vi "Try Beta Version of CSMF.vi"() -> ()   [LabVIEW 2017]
uses:
  <vilib>/JKI/VIPM API/command-line/support/Library Contents Cluster_vipm_api.ctl
  _Try Beta Version of CSMF/_Try Beta Version of CSMF.lvlib
  <vilib>/JKI/VIPM API/VIPM API_vipm_api.lvlib
panel:
  out "Next Actions":string
  out "Information":string
  # "Warning: You should login VIPM and change it to community/Pro edtion firstly."
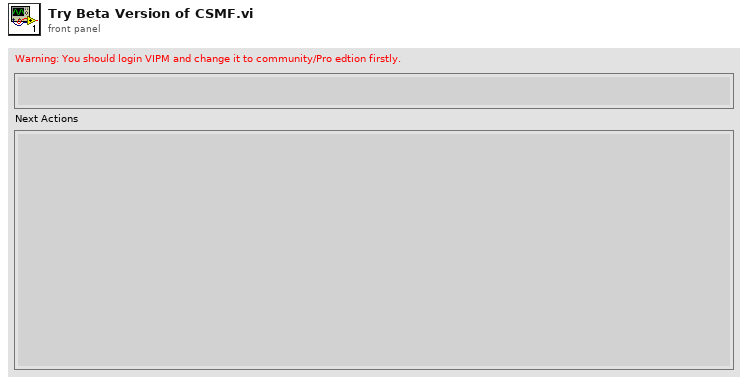
[diagram p1: front panel]
types:
  T1 = enum32{"Invalid", "Standard", "Closed", "Hidden", "Minimized", "Maximized"}
  T2 = enum32{"invalid app kind", "Development System", "Run Time System", "Student Edition", "Embedded LabVIEW", "Evaluation", "Custom"}
  T3 = enum16{"open", "replace", "create", "open or create", "replace or create", "replace or create with confirmation"}
  T4 = typedef "VIPM API_vipm_api.lvlib/Library Contents Cluster_vipm_api.ctl" = cluster{"Package Name":string, "Version":string, "Display Name":string, "Repository Name":string, "Company Name":string, "License Type":string, "Installed":bool, "Deprecated":bool, "Dependency or Conflict Problem":bool, "Downloaded":bool}
  T5 = cluster{"Core":cluster{"Current VI Reference":refnum<vi>, "Close Panel on Exit?":bool}, "ftpInfo":cluster{"address":string, "remote port (21)":u16, "userName":string, "passWord":string}, "CSMF":string[], "Library[]":T4[], "CSMFTempPath":path[]}
  T6 = cluster{"address":string, "remote port (21)":u16, "userName":string, "passWord":string}
  T7 = cluster{"Current VI Reference":refnum<vi>, "Close Panel on Exit?":bool}
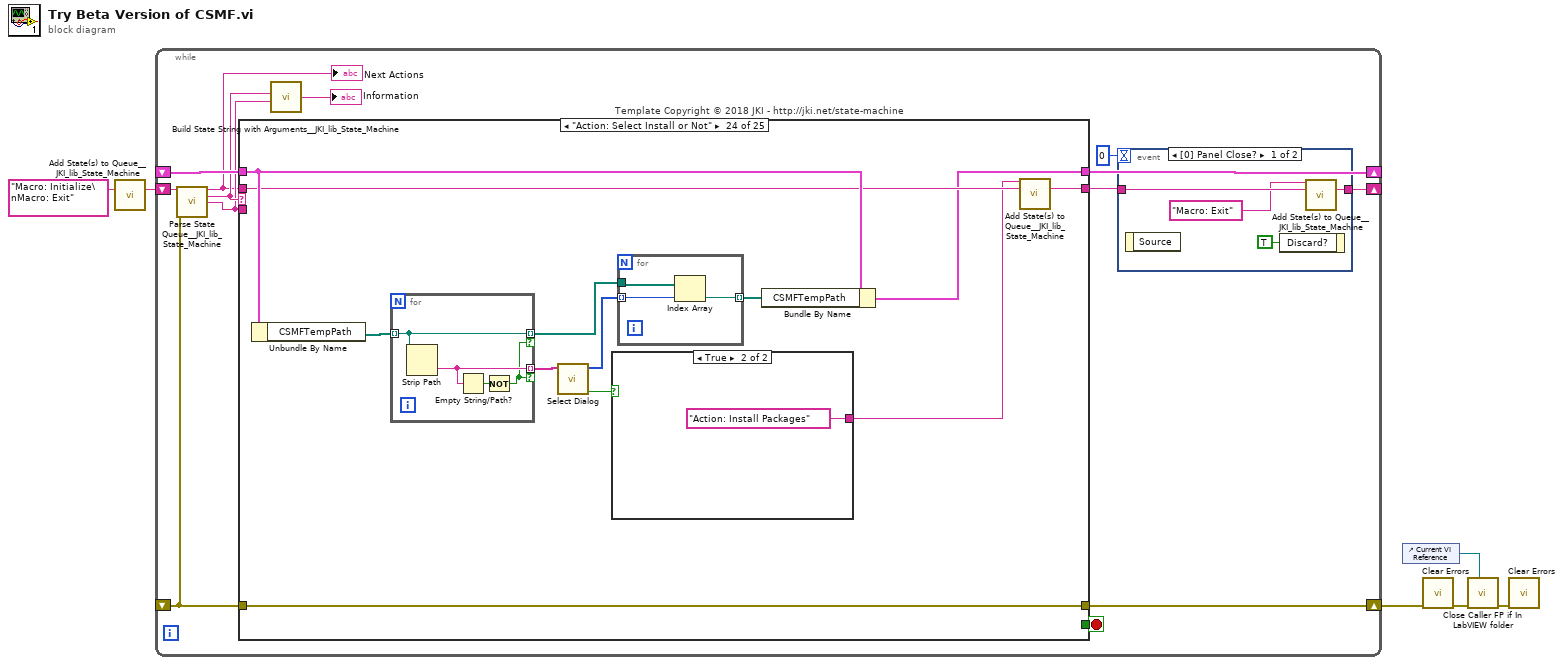
[diagram p0: block diagram]
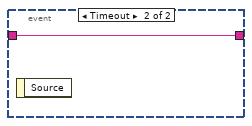
[diagram p2: hidden frame]
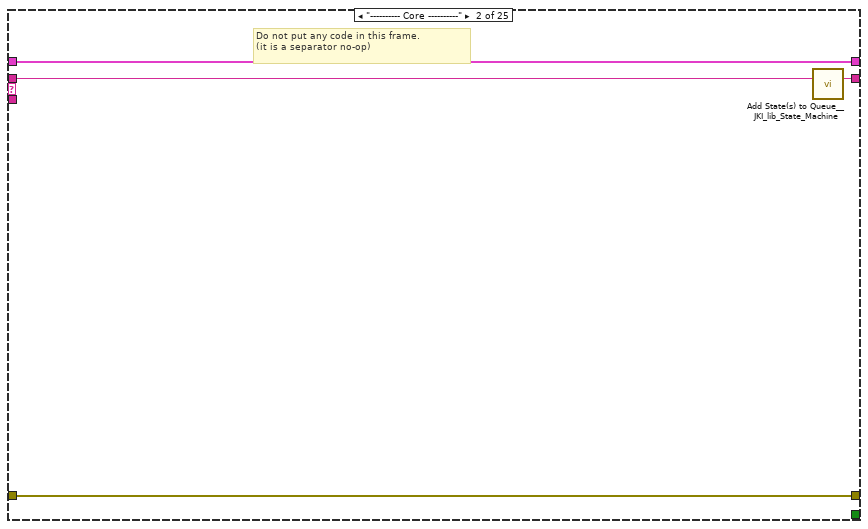
[diagram p4: hidden frame]
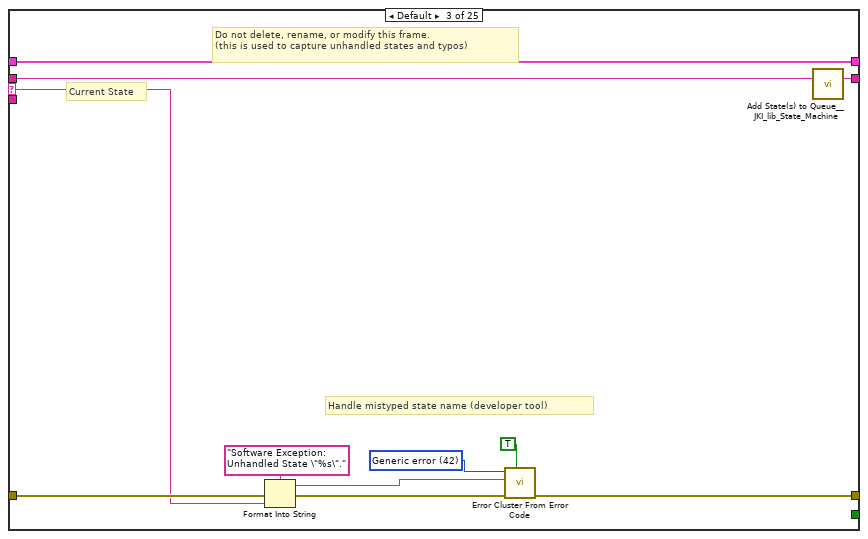
[diagram p5: hidden frame]
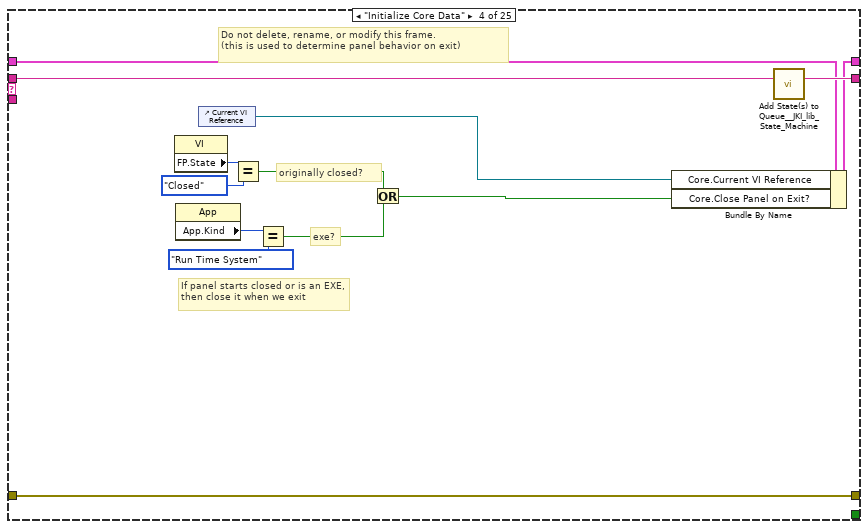
[diagram p6: hidden frame]
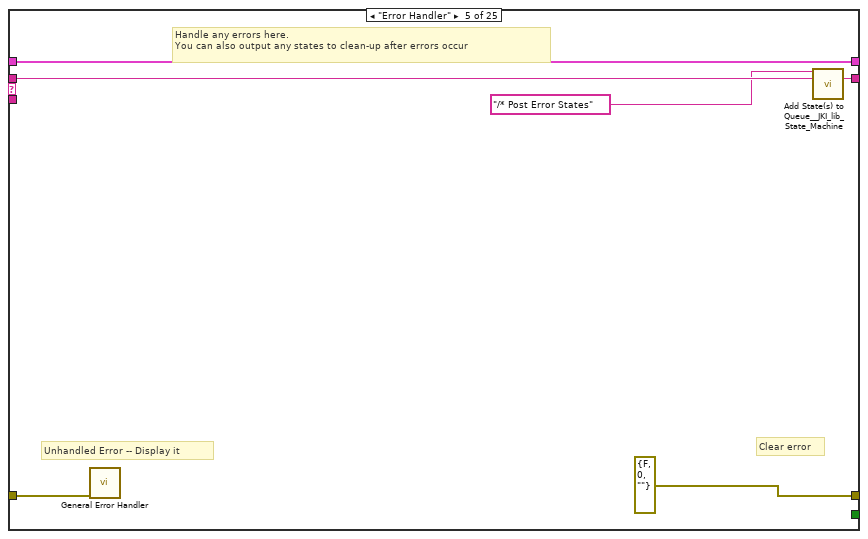
[diagram p7: hidden frame]
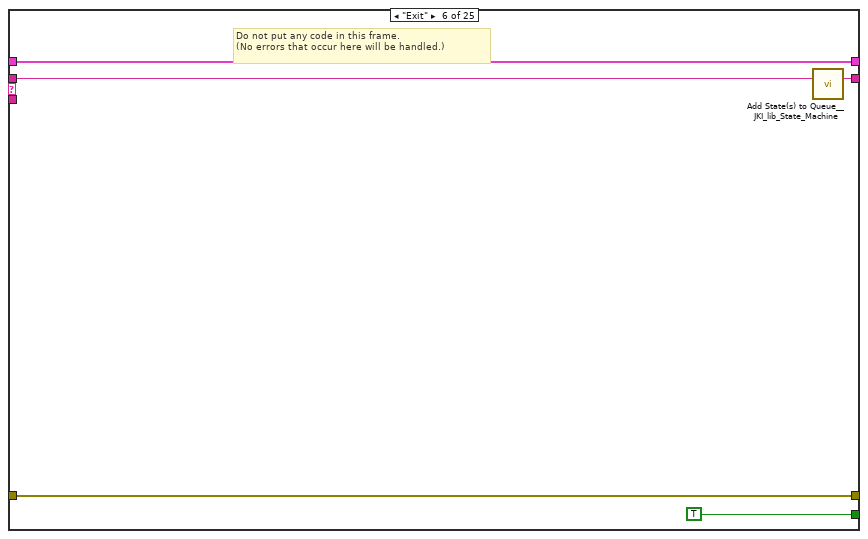
[diagram p8: hidden frame]
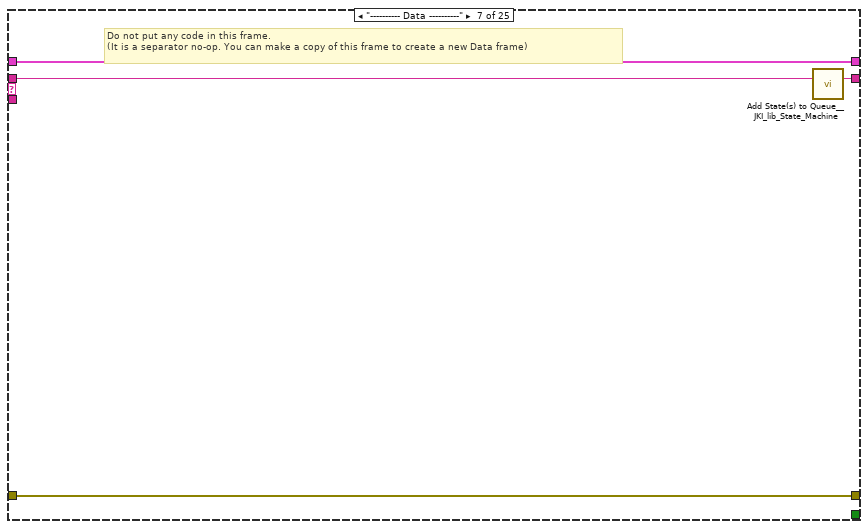
[diagram p9: hidden frame]
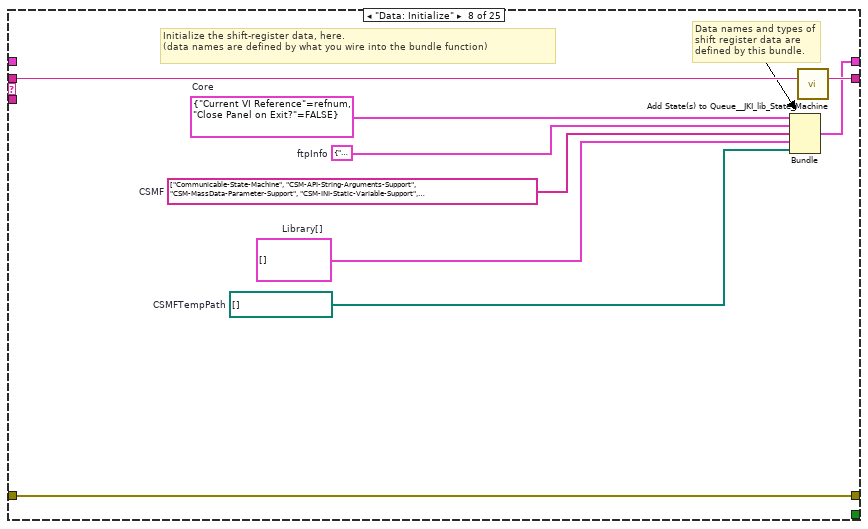
[diagram p10: hidden frame]
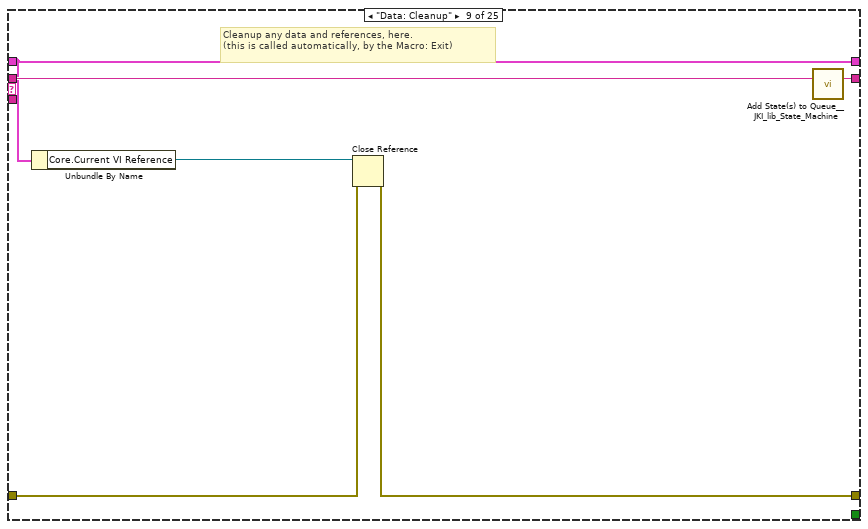
[diagram p11: hidden frame]
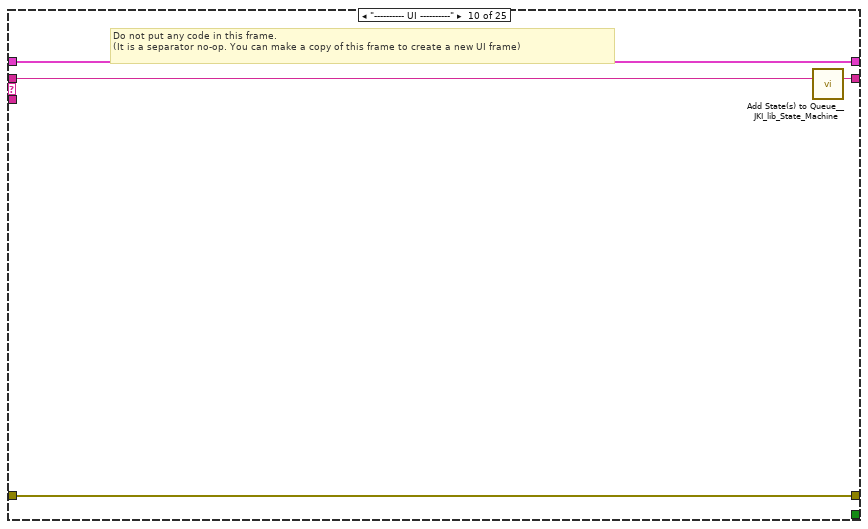
[diagram p12: hidden frame]
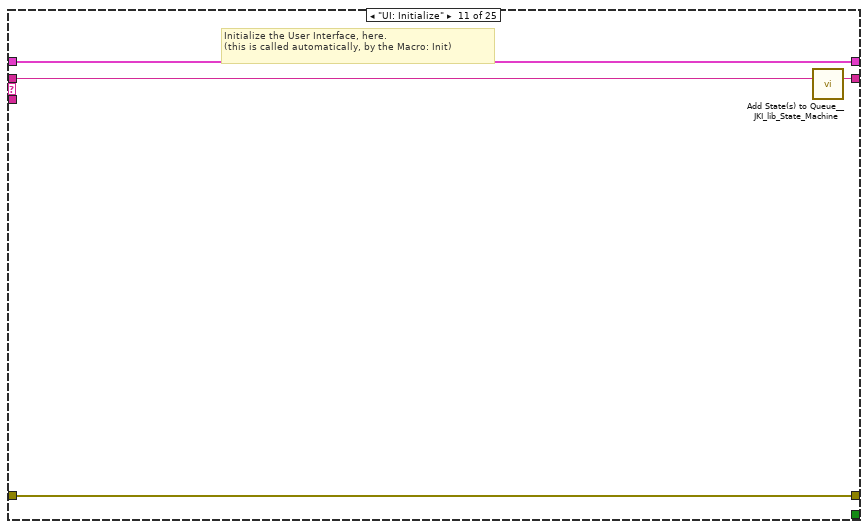
[diagram p13: hidden frame]
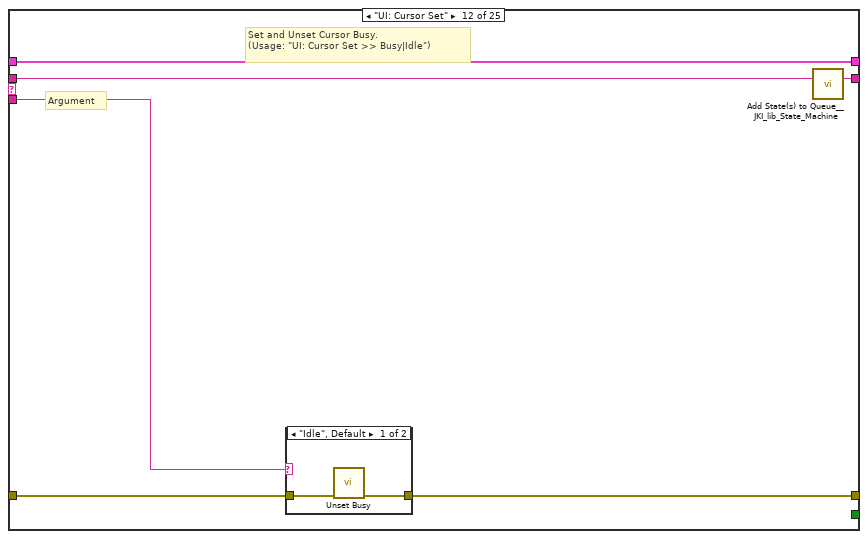
[diagram p14: hidden frame]
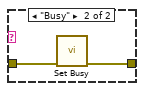
[diagram p15: hidden frame]
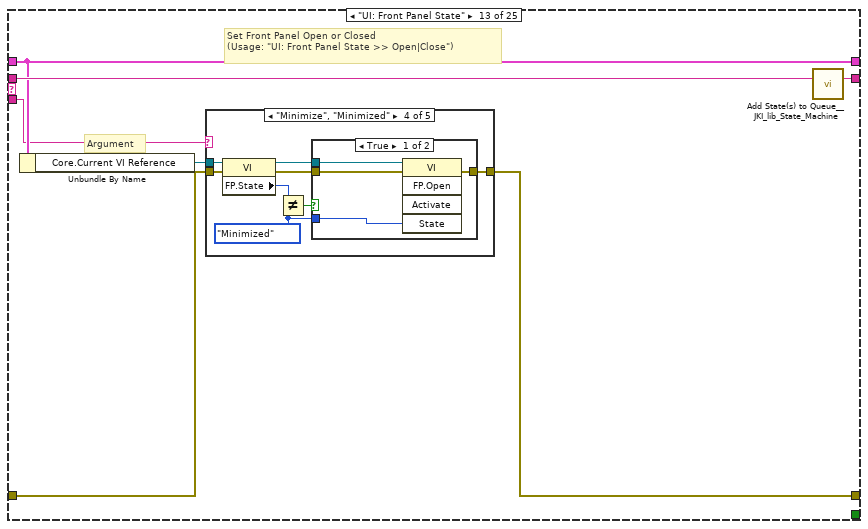
[diagram p16: hidden frame]
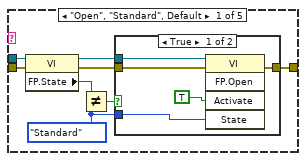
[diagram p17: hidden frame]
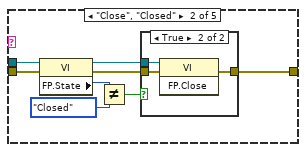
[diagram p19: hidden frame]
diagram:
  n1 = call <vilib>:"Add State(s) to Queue__JKI_lib_State_Machine.vi"("State(s) in (\"\")"="Macro: Initialize\nMacro: Exit") -> ("States Out"=w3:string)  [unwired: 14 in]
  n2 = while {
    shift-right: [w16] -> _
    shift-left: _ -> [w15]
    shift-right: [w18] -> w2
    shift-left: _ -> [w14]
    shift-right: [w8] -> _
    shift-left: w3 -> [w19]
    stop <- w17 stop-if-true
    # "Template Copyright © 2018 JKI - http://jki.net/state-machine"
    n3 = call <vilib>:"Parse State Queue__JKI_lib_State_Machine.vi"("State Queue"=w19, "Error In (no error)"=w14) -> ("Remaining States"=w10:string, "Current State"=w13:string, "Arguments"=w11:string)  [unwired: 11 in]
    "Next Actions" <- w10
    n4 = case shown="\"Action: Select Install or Not\"" w13 {
      selector: w13 -> [_ _ w32 _ _ _ _ _ _ _ _ _ _ _ _ _ _ _ _ _ _ _ _ _ _]
      tunnel: w10 -> [w27 w31 w36 w55 w61 w66 w70 w79 w85 w89 w93 w99 w110 w179 w184 w189 w207 w211 w225 w231 w241 w247 w254 w263 w287]
      tunnel: w11 -> [_ _ _ _ _ _ _ _ _ _ _ w94 w104 _ _ _ _ _ _ _ w238 _ _ _ _]
      tunnel: w15 -> [w25 w28 w34 w48 w58 w64 w67 _ w80 w86 w91 w97 w106 w176 w181 w186 w204 w208 w216 w228 w240 w250 w253 w265 w286]
      tunnel: [w26 w29 w38 w52 errorcluster {"status"=FALSE, "code"=0, "source"=""} ("error out") w63 w68 w76 w81 w87 w90 w95 w107 w177 w182 w192 w205 w209 w223 w229 w234 w249 w251 w266 w275] -> w18
      tunnel: w14 -> [w26 w29 w37 w52 w57 w63 w68 w76 w82 w87 w90 w96 w108 w177 w182 w192 w205 w209 w223 w229 _ _ _ w266 _]
      tunnel: [w27 w30 w35 w54 w60 w65 w69 w78 w84 w88 w92 w98 w109 w178 w183 w190 w206 w210 w224 w230 w241 w248 w254 w264 w287] -> w9
      tunnel: [_ _ _ _ _ TRUE _ _ _ _ _ _ _ _ _ _ _ _ _ _ _ _ _ _ _] -> w17
      tunnel: [w25 w28 w34 w53 w58 w64 w67 w77 w80 w86 w91 w97 w106 w176 w181 w186 w204 w208 w214 w227 w236 w250 w253 w259 w278] -> w16
      frame "", "Event Structure", "Idle" {
        # "executes when the state queue is empty"
      }
      frame "---------- Core ----------" {
        # "Do not put any code in this frame.\n(it is a separator no-op)"
        n5 = call <vilib>:"Add State(s) to Queue__JKI_lib_State_Machine.vi"("State(s) in (\"\")"=w31) -> ("States Out"=w30:string)  [unwired: 14 in]
      }
      frame Default {
        w41 = 42 items=["No error", "Argument error", "Memory is full", "Out of zone", "End of file", "File already open", "Generic file I/O error", "File not found", "File permission error", "Disk is full", "Duplicate path", "Too many files open", "System feature not enabled", "Resource file not found", "Cannot add resource", "Resource not found", "Image not found", "Image memory error", "Pen does not exist", "Config type invalid", "Config token not found", "Config parse error", "Config memory error", "Bad external code format", "Bad external code offset", "External code not present", "Null window", "Destroy window error", "Null menu", "Print aborted", "Bad print record", "Print driver error", "Windows error during printing", "Memory error during printing", "Print dialog error", "Generic print error", "Invalid device refnum", "Device not found", "Device parameter error", "Device unit error", "Cannot open device", "Device call aborted", "Generic error", "Cancelled by user", "Object ID too low", "Object ID too high", "Object not in heap", "Unknown heap", "Unknown object (invalid DefProc)", "Unknown object (DefProc not in table)", "Message out of range", "Invalid (null) method", "Unknown message", "Manager call not supported", "Bad address", "Network operation in progress", "Network operation timed out", "Connection is busy", "Network attribute not supported", "Network error", "Address in use", "System out of memory", "Connection aborted", "Connection refused", "Not connected", "Already connected", "Connection closed", "Initialization error (interapplication manager)", "Bad occurrence", "Wait on unbound occurrence handler", "Occurrence queue overflow", "Datalog type conflict", "Unused", "Unrecognized type (interapplication manager)", "Memory corrupt", "Failed to make temporary DLL", "Old CIN version", "Drag socket not found", "Failed to load drop-object", "Failed to register OLE object", "Failed to release OLE object", "Format specifier type mismatch", "Unknown format specifier", "Too few format specifiers", "Too many format specifiers", "Scan failed", "Newer CIN version", "Error converting to variant", "Runtime menu error", "Password tampered", "Variant attribute not found", "Incompatible variant data type", "Event data is not available", "Event Store is not present", "Occurrence is not found", "Event Queue is not created", "Event info is not available", "Refnum passed is NULL", "Error retrieving Class GUID", "Error retrieving CoClass GUID", "Error retrieving TypeLib GUID.", "Bad built application magic bytes.", "Specific driver is different from the specific driver associated with the Logical Name.", "There is no session opened to the class driver.", "Max Error", "MAX - Error with config objects", "MAX - Error loading configuration", "MAX - Group not supported"]
        # "Current State"
        # "Do not delete, rename, or modify this frame.\n(this is used to capture unhandled states and typos)"
        # "Handle mistyped state name (developer tool)"
        n6 = Format Into String(format string="Software Exception: Unhandled State \"%s\"." ("message"), error in=w37, w32) -> (resulting string=w40:string, error out=w39:errorcluster)  [unwired: 1 in]
        n7 = call <vilib>:"Error Cluster From Error Code.vi"("show call chain? (False)"=TRUE, "error in (no error)"=w39, "error message (\"\")"=w40, "error code (0)"=w41) -> ("error out"=w38:errorcluster)  [unwired: 5 in]
        n8 = call <vilib>:"Add State(s) to Queue__JKI_lib_State_Machine.vi"("State(s) in (\"\")"=w36) -> ("States Out"=w35:string)  [unwired: 14 in]
      }
      frame "Initialize Core Data" {
        # "Do not delete, rename, or modify this frame.\n(this is used to determine panel behavior on exit)"
        # "originally closed?"
        # "exe?"
        # "If panel starts closed or is an EXE, then close it when we exit"
        n9 = property class="VI"() -> ("FP.State"=w45:T1)  [unwired: 2 in, 2 out]
        n10 = property class="App"() -> ("App.Kind"=w51:T2)  [unwired: 2 in, 2 out]
        n11 = control-ref of="Current VI Reference"() -> (w46:refnum<vi>)
        n12 = Equal?(x=w45, y=T1."Closed" ("Front Panel Window:State")) -> (x = y?=w43:bool)
        n13 = Equal?(x=w51, y=T2."Run Time System" ("Application:Kind")) -> (x = y?=w49:bool)
        n14 = Or(x=w43, y=w49) -> (x .or. y?=w47:bool)
        n15 = Bundle By Name(cluster=w48, "Core.Current VI Reference"=w46, "Core.Close Panel on Exit?"=w47) -> (w53:T5)
        n16 = call <vilib>:"Add State(s) to Queue__JKI_lib_State_Machine.vi"("State(s) in (\"\")"=w55) -> ("States Out"=w54:string)  [unwired: 14 in]
      }
      frame "Error Handler" {
        # "Unhandled Error -- Display it"
        # "Handle any errors here.\nYou can also output any states to clean-up after errors occur"
        # "Clear error"
        n17 = call <vilib>:"General Error Handler.vi"("error in (no error)"=w57) -> ()  [unwired: 10 in, 5 out]
        n18 = call <vilib>:"Add State(s) to Queue__JKI_lib_State_Machine.vi"("State(s) in Front (\"\")"="/* Post Error States", "State(s) in (\"\")"=w61) -> ("States Out"=w60:string)  [unwired: 13 in]
      }
      frame "Exit" {
        # "Do not put any code in this frame.\n(No errors that occur here will be handled.)"
        n19 = call <vilib>:"Add State(s) to Queue__JKI_lib_State_Machine.vi"("State(s) in (\"\")"=w66) -> ("States Out"=w65:string)  [unwired: 14 in]
      }
      frame "---------- Data ----------" {
        # "Do not put any code in this frame.\n(It is a separator no-op. You can make a copy of this frame to create a new Data frame)"
        n20 = call <vilib>:"Add State(s) to Queue__JKI_lib_State_Machine.vi"("State(s) in (\"\")"=w70) -> ("States Out"=w69:string)  [unwired: 14 in]
      }
      frame "Data: Initialize" {
        w71 = path[] []  # CSMFTempPath
        w72 = T4[] []  # Library[]
        w73 = string[] ["Communicable-State-Machine", "CSM-API-String-Arguments-Support", "CSM-MassData-Parameter-Support", "CSM-INI-Static-Variable-Support", "CSM-Continuous-Meausrement-and-Logging", "CSM-TCP-Router-App", "CSM-Mermaid-Plugin"]  # CSMF
        w74 = T6 {"address"="vipm.nevstop.top", "remote port (21)"=1986, "userName"="", "passWord"=""}  # ftpInfo
        w75 = T7 {"Current VI Reference"=refnum, "Close Panel on Exit?"=FALSE}  # Core
        # "Data names and types of shift register data are defined by this bundle."
        # "Initialize the shift-register data, here.\n(data names are defined by what you wire into the bundle function)"
        n21 = Bundle("Core"=w75, "ftpInfo"=w74, "CSMF"=w73, "Library[]"=w72, "CSMFTempPath"=w71) -> (w77:T5)  [unwired: 1 in]
        n22 = call <vilib>:"Add State(s) to Queue__JKI_lib_State_Machine.vi"("State(s) in (\"\")"=w79) -> ("States Out"=w78:string)  [unwired: 14 in]
      }
      frame "Data: Cleanup" {
        # "Cleanup any data and references, here.\n(this is called automatically, by the Macro: Exit)"
        n23 = Unbundle By Name(w80) -> ("Core.Current VI Reference"=w83:refnum<vi>)
        n24 = Close Reference(reference=w83, error in (no error)=w82) -> (error out=w81:errorcluster)
        n25 = call <vilib>:"Add State(s) to Queue__JKI_lib_State_Machine.vi"("State(s) in (\"\")"=w85) -> ("States Out"=w84:string)  [unwired: 14 in]
      }
      frame "---------- UI ----------" {
        # "Do not put any code in this frame.\n(It is a separator no-op. You can make a copy of this frame to create a new UI frame)"
        n26 = call <vilib>:"Add State(s) to Queue__JKI_lib_State_Machine.vi"("State(s) in (\"\")"=w89) -> ("States Out"=w88:string)  [unwired: 14 in]
      }
      frame "UI: Initialize" {
        # "Initialize the User Interface, here.\n(this is called automatically, by the Macro: Init)"
        n27 = call <vilib>:"Add State(s) to Queue__JKI_lib_State_Machine.vi"("State(s) in (\"\")"=w93) -> ("States Out"=w92:string)  [unwired: 14 in]
      }
      frame "UI: Cursor Set" {
        # "Argument"
        # "Set and Unset Cursor Busy.\n(Usage: \"UI: Cursor Set >> Busy|Idle\")"
        n28 = case shown="\"Idle\", Default" w94 {
          tunnel: w96 -> [w101 w103]
          tunnel: [w100 w102] -> w95
          frame "Idle", Default {
            n29 = call <vilib>:"Unset Busy.vi"("error in (no error)"=w101) -> ("error out"=w100:errorcluster)  [unwired: 10 in]
          }
          frame "Busy" {
            n30 = call <vilib>:"Set Busy.vi"("error in (no error)"=w103) -> ("error out"=w102:errorcluster)  [unwired: 9 in, 1 out]
          }
        }
        n31 = call <vilib>:"Add State(s) to Queue__JKI_lib_State_Machine.vi"("State(s) in (\"\")"=w99) -> ("States Out"=w98:string)  [unwired: 14 in]
      }
      frame "UI: Front Panel State" {
        # "Argument"
        # "Set Front Panel Open or Closed\n(Usage: \"UI: Front Panel State >> Open|Close\")"
        n32 = Unbundle By Name(w106) -> ("Core.Current VI Reference"=w105:refnum<vi>)
        n33 = case shown="\"Minimize\", \"Minimized\"" w104 {
          tunnel: w108 -> [w116 w131 w142 w155 w168]
          tunnel: [w118 w132 w144 w157 w170] -> w107
          tunnel: w105 -> [w117 w129 w143 w156 w169]
          frame "Open", "Standard", Default {
            w111 = T1."Standard" ("State")
            n34 = property class="VI"(reference=w117, error in=w116) -> (reference out=w114:refnum<vi>, error out=w115:errorcluster, "FP.State"=w113:T1)
            n35 = Not Equal?(x=w113, y=w111) -> (x != y?=w112:bool)
            n36 = case shown="True" w112 {
              tunnel: [w122 w124] -> w118
              tunnel: w115 -> [w121 w124]
              tunnel: w114 -> [w120 _]
              tunnel: w111 -> [w119 _]
              frame True {
                n37 = invoke class="VI" method="FP.Open"(reference=w120, error in=w121, "Activate"=TRUE, "State"=w119) -> (error out=w122:errorcluster)  [unwired: 1 in, 4 out]
              }
              frame False {
              }
            }
          }
          frame "Close", "Closed" {
            n38 = property class="VI"(reference=w129, error in=w131) -> (reference out=w128:refnum<vi>, error out=w130:errorcluster, "FP.State"=w126:T1)
            n39 = Not Equal?(x=w126, y=T1."Closed" ("Front Panel Window:State")) -> (x != y?=w125:bool)
            n40 = case shown="True" w125 {
              tunnel: [w133 w136] -> w132
              tunnel: w130 -> [w133 w135]
              tunnel: w128 -> [_ w134]
              frame False {
              }
              frame True {
                n41 = invoke class="VI" method="FP.Close"(reference=w134, error in=w135) -> (error out=w136:errorcluster)  [unwired: 1 in, 2 out]
              }
            }
          }
          frame "Hidden", "Hide" {
            w137 = T1."Hidden" ("State")
            n42 = property class="VI"(reference=w143, error in=w142) -> (reference out=w140:refnum<vi>, error out=w141:errorcluster, "FP.State"=w139:T1)
            n43 = Not Equal?(x=w139, y=w137) -> (x != y?=w138:bool)
            n44 = case shown="True" w138 {
              tunnel: [w148 w149] -> w144
              tunnel: w141 -> [w147 w149]
              tunnel: w140 -> [w146 _]
              tunnel: w137 -> [w145 _]
              frame True {
                n45 = invoke class="VI" method="FP.Open"(reference=w146, error in=w147, "State"=w145) -> (error out=w148:errorcluster)  [unwired: 2 in, 4 out]
              }
              frame False {
              }
            }
          }
          frame "Minimize", "Minimized" {
            w150 = T1."Minimized" ("State")
            n46 = property class="VI"(reference=w156, error in=w155) -> (reference out=w153:refnum<vi>, error out=w154:errorcluster, "FP.State"=w152:T1)
            n47 = Not Equal?(x=w152, y=w150) -> (x != y?=w151:bool)
            n48 = case shown="True" w151 {
              tunnel: [w161 w162] -> w157
              tunnel: w154 -> [w160 w162]
              tunnel: w153 -> [w159 _]
              tunnel: w150 -> [w158 _]
              frame True {
                n49 = invoke class="VI" method="FP.Open"(reference=w159, error in=w160, "State"=w158) -> (error out=w161:errorcluster)  [unwired: 2 in, 4 out]
              }
              frame False {
              }
            }
          }
          frame "Maximize", "Maximized" {
            w163 = T1."Maximized" ("State")
            n50 = property class="VI"(reference=w169, error in=w168) -> (reference out=w166:refnum<vi>, error out=w167:errorcluster, "FP.State"=w165:T1)
            n51 = Not Equal?(x=w165, y=w163) -> (x != y?=w164:bool)
            n52 = case shown="True" w164 {
              tunnel: [w174 w175] -> w170
              tunnel: w167 -> [w173 w175]
              tunnel: w166 -> [w172 _]
              tunnel: w163 -> [w171 _]
              frame True {
                n53 = invoke class="VI" method="FP.Open"(reference=w172, error in=w173, "State"=w171) -> (error out=w174:errorcluster)  [unwired: 2 in, 4 out]
              }
              frame False {
              }
            }
          }
        }
        n54 = call <vilib>:"Add State(s) to Queue__JKI_lib_State_Machine.vi"("State(s) in (\"\")"=w110) -> ("States Out"=w109:string)  [unwired: 14 in]
      }
      frame "---------- Macro ----------" {
        # "Do not put any code in this frame.\n(It is a separator no-op. You can make a copy of this frame to create a new Macro frame)"
        n55 = call <vilib>:"Add State(s) to Queue__JKI_lib_State_Machine.vi"("State(s) in (\"\")"=w179) -> ("States Out"=w178:string)  [unwired: 14 in]
      }
      frame "Macro: Initialize" {
        w180 = "Data: Initialize\nInitialize Core Data\nUI: Initialize\nUI: Front Panel State >> Open\nAction: List FTP Information\nAction: List CSM Framework Pacakges\nAction: Check Package List\nMacro: Action: Check CSMF Newest Package in FTP\nAction: Select Install or Not"  # Data: Initialize Initialize Core Data UI: Initialize UI: Front Panel State >> Open Action: List FTP Information Action: List CSM Framework Pacakges Action: Check Package List Macro: Action: Check CSMF Newest Package in FTP Action: Select Install or Not
        n56 = call <vilib>:"Add State(s) to Queue__JKI_lib_State_Machine.vi"("State(s) in Front (\"\")"=w180, "State(s) in (\"\")"=w184) -> ("States Out"=w183:string)  [unwired: 13 in]
      }
      frame "Macro: Action: Check CSMF Newest Package in FTP" {
        n57 = Unbundle By Name(w186) -> ("CSMF"=w185:string[])
        n58 = for {
          tunnel: "Action: Check CSMF Newest Package in FTP" ("State") -> [w197]
          shift-right: [w196] -> w187
          shift-left: "" ("States Out") -> [w194]
          tunnel: w185 -> [w195] mode=indexing
          n59 = call <vilib>:"Build State String with Arguments__JKI_lib_State_Machine.vi"("Arguments (\"\")"=w195, "State"=w197) -> ("State with Arguments"=w193:string)  [unwired: 4 in]
          n60 = call <vilib>:"Add State(s) to Queue__JKI_lib_State_Machine.vi"("State(s) in Front (\"\")"=w194, "State(s) in (\"\")"=w193) -> ("States Out"=w196:string)  [unwired: 13 in]
        }
        n61 = call <vilib>:"Add State(s) to Queue__JKI_lib_State_Machine.vi"("State(s) in Front (\"\")"=w187, "State(s) in (\"\")"=w189) -> ("States Out"=w190:string)  [unwired: 13 in]
      }
      frame "Macro: Exit" {
        # "Exit Macro\n(This is called once, when the VI exits)"
        n62 = Unbundle By Name(w204) -> ("Core.Close Panel on Exit?"=w203:bool)
        n63 = Select(t="UI: Front Panel State >> Close", s=w203, f="") -> (s? t:f=w200:string)
        n64 = call <vilib>:"Add State(s) to Queue__JKI_lib_State_Machine.vi"("State(s) in (\"\")"=w200, "State(s) at Back (\"\")"="Data: Cleanup\nExit") -> ("States Out"=w198:string)  [unwired: 13 in]
        n65 = call <vilib>:"Add State(s) to Queue__JKI_lib_State_Machine.vi"("State(s) in Front (\"\")"=w198, "State(s) in (\"\")"=w207) -> ("States Out"=w206:string)  [unwired: 13 in]
      }
      frame "---------- Action ----------" {
        # "Template Separator\n(You can make a copy of, or modify, this frame)"
        n66 = call <vilib>:"Add State(s) to Queue__JKI_lib_State_Machine.vi"("State(s) in (\"\")"=w211) -> ("States Out"=w210:string)  [unwired: 14 in]
      }
      frame "Action: List FTP Information" {
        n67 = Index Array(array=string[] ["vipm.nevstop.top", "1986", "anonymous", ""] ("CommandLine")) -> (element #1=w222:string, element #2=w221:string, element #3=w218:string, element #4=w219:string)  [unwired: 5 in, 1 out]
        n68 = Equal?(x=w218, y="anonymous") -> ()  [unwired: 1 out]
        n69 = Decimal String To Number(string=w221) -> (number=w220:i32)  [unwired: 2 in, 1 out]
        n70 = Unbundle By Name(w216) -> ("ftpInfo"=w215:T6)
        n71 = Bundle By Name(cluster=w215, "address"=w222, "remote port (21)"=w220, "userName"=w218, "passWord"=w219) -> (w213:T6)
        n72 = Bundle By Name(cluster=w216, "ftpInfo"=w213) -> (w214:T5)
        n73 = call <vilib>:"Add State(s) to Queue__JKI_lib_State_Machine.vi"("State(s) in (\"\")"=w225) -> ("States Out"=w224:string)  [unwired: 14 in]
      }
      frame "Action: List CSM Framework Pacakges" {
        n74 = Bundle By Name(cluster=w228, "CSMF"=string[] ["Communicable-State-Machine", "CSM-API-String-Arguments-Support", "CSM-MassData-Parameter-Support", "CSM-INI-Static-Variable-Support", "CSM-Continuous-Meausrement-and-Logging", "CSM-TCP-Router-App", "CSM-Mermaid-Plugin"] ("element")) -> (w227:T5)
        n75 = call <vilib>:"Add State(s) to Queue__JKI_lib_State_Machine.vi"("State(s) in (\"\")"=w231) -> ("States Out"=w230:string)  [unwired: 14 in]
      }
      frame "Action: Check CSMF Newest Package in FTP" {
        n76 = Unbundle By Name(w240) -> ("CSMFTempPath"=w237:path[], "ftpInfo"=w239:T6)
        n77 = call "DownloadPackageFromNevstopFTP.vi"("ftp"=w239, "CommandLine"=w238) -> ("error out"=w234:errorcluster, "localdir"=w233:path)  [unwired: 7 in, 1 out]
        n78 = Empty String/Path?(string/path=w233) -> (empty?=w232:bool)
        n79 = case shown="False" w232 {
          tunnel: w237 -> [w244 w245]
          tunnel: [w243 w245] -> w235
          tunnel: w233 -> [w242 _]
          frame False {
            n80 = Build Array (concatenate)(w244, w242) -> (w243:path[])
          }
          frame True {
          }
        }
        n81 = Bundle By Name(cluster=w240, "CSMFTempPath"=w235) -> (w236:T5)
      }
      frame "Action: Install Packages" {
        n82 = Unbundle By Name(w250) -> ("CSMFTempPath"=w246:path[])
        n83 = call "vipm_InstallPackages.vi"("CommandLine"=w246) -> ("error out"=w249:errorcluster)  [unwired: 8 in, 2 out]
        n84 = call <vilib>:"Add State(s) to Queue__JKI_lib_State_Machine.vi"("State(s) in (\"\")"=w247) -> ("States Out"=w248:string)  [unwired: 14 in]
      }
      frame "Action: Switch to Current Version in VIPM" {
        n85 = call "vipm_target_version.vi"() -> ("vipm Taget version"=w252:string)  [unwired: 11 in]
        n86 = call <vilib>:"Switch Target_vipm_api.vi"("LabVIEW Version"=w252) -> ("error out"=w251:errorcluster)  [unwired: 10 in]
      }
      frame "Action: Select Install or Not" {
        n87 = Unbundle By Name(w265) -> ("CSMFTempPath"=w256:path[])
        n88 = for {
          tunnel: w256 -> [w273] mode=indexing
          tunnel: [w271] -> w261 mode=indexing if=w270
          tunnel: [w273] -> w255 mode=indexing if=w270
          n89 = Strip Path(path=w273) -> (name=w271:string)  [unwired: 1 out]
          n90 = Empty String/Path?(string/path=w271) -> (empty?=w272:bool)
          n91 = Not(x=w272) -> (.not. x?=w270:bool)
        }
        n92 = call "Select Dialog.vi"("Item Names"=w261) -> ("Install?"=w260:bool, "candidates out"=w258:i32[])  [unwired: 9 in]
        n93 = case shown="True" w260 {
          tunnel: [_ "Action: Install Packages" ("State(s) in Front (\"\")")] -> w262
          frame False {
          }
          frame True {
          }
        }
        n94 = for {
          tunnel: w255 -> [w269]
          tunnel: w258 -> [w268] mode=indexing
          tunnel: [w267] -> w257 mode=indexing
          n95 = Index Array(array=w269, index=w268) -> (element=w267:path)
        }
        n96 = Bundle By Name(cluster=w265, "CSMFTempPath"=w257) -> (w259:T5)
        n97 = call <vilib>:"Add State(s) to Queue__JKI_lib_State_Machine.vi"("State(s) in Front (\"\")"=w262, "State(s) in (\"\")"=w263) -> ("States Out"=w264:string)  [unwired: 13 in]
      }
      frame "Action: Check Package List" {
        n98 = Current VI's Path() -> (path=w280:path)
        n99 = Unbundle By Name(w286) -> ("CSMF"=w277:string[])
        n100 = Strip Path(path=w280) -> (stripped path=w281:path)  [unwired: 1 out]
        n101 = Build Path(base path=w281, name or relative path="CSMF Package List.txt") -> (appended path=w282:path)
        n102 = call <vilib>:"Check if File or Folder Exists.vi"("path"=w282) -> ("error out"=w285:errorcluster, "file or folder exists?"=w284:bool, "dup path"=w283:path)  [unwired: 8 in]
        n103 = case shown="True" w284 {
          tunnel: w283 -> [w295 w315]
          tunnel: w285 -> [w294 w309]
          tunnel: w277 -> [w290 _]
          tunnel: [w290 w301] -> w276
          tunnel: [w288 w307] -> w275
          frame False {
            n104 = call "1D Array to String.vi"("delimiter (Tab)"="\r", "Array of Strings"=w290) -> ("delimited string"=w291:string)  [unwired: 9 in]
            n105 = call <vilib>:"Trim Whitespace.vi"("string"=w291) -> ("trimmed string"=w289:string)  [unwired: 1 in]
            n106 = Open/Create/Replace File(file path (use dialog)=w295, error in=w294, operation (0:open)=T3."replace or create") -> (refnum out=w298:refnum<file>, error out=w299:errorcluster)  [unwired: 3 in, 1 out]
            n107 = Write to Text File(file (use dialog)=w298, text=w289, error in=w299) -> (refnum out=w296:refnum<file>, error out=w297:errorcluster)  [unwired: 1 in, 1 out]
            n108 = Close File(refnum=w296, error in=w297) -> (error out=w288:errorcluster)  [unwired: 1 out]
          }
          frame True {
            w302 = "\n" ("delimiter (Tab)")
            n109 = Open/Create/Replace File(file path (use dialog)=w315, error in=w309, operation (0:open)=T3."open") -> (refnum out=w313:refnum<file>, error out=w314:errorcluster)  [unwired: 3 in, 1 out]
            n110 = Read from Text File(file (use dialog)=w313, error in=w314) -> (refnum out=w311:refnum<file>, text=w308:string, error out=w312:errorcluster)  [unwired: 2 in, 1 out]
            n111 = call <vilib>:"Trim Whitespace.vi"("string"=w308) -> ("trimmed string"=w306:string)  [unwired: 1 in]
            n112 = Close File(refnum=w311, error in=w312) -> (error out=w307:errorcluster)  [unwired: 1 out]
            n113 = Search and Replace String(replace all?=TRUE ("replace all? (F)"), input string=w306, search string="\r\n", replace string=w302) -> (result string=w305:string)  [unwired: 4 in, 3 out]
            n114 = call "String to 1D Array.vi"("delimiter (Tab)"=w302, "string"=w305) -> ("Array of Strings"=w300:string[])  [unwired: 9 in]
            n115 = for {
              tunnel: [w319] -> w301 mode=indexing if=w316
              tunnel: w300 -> [w319] mode=indexing
              n116 = Match Pattern(string=w319, regular expression="^[#]") -> (offset past match=w317:i32)  [unwired: 1 in, 3 out]
              n117 = Less Than 0?(x=w317) -> (x < 0?=w316:bool)
            }
          }
        }
        n118 = Bundle By Name(cluster=w286, "CSMF"=w276) -> (w278:T5)
      }
    }
    n119 = call <vilib>:"Build State String with Arguments__JKI_lib_State_Machine.vi"("Arguments (\"\")"=w11, "State"=w13) -> ("State with Arguments"=→"Information":string)  [unwired: 4 in]
    n120 = event shown="[0] Panel Close?" {
      selector: _ -> [_ _]
      dyn-events: _ -> [_ _]
      timeout: 0 -> [_ _]
      tunnel: w9 -> [w23 w24]
      tunnel: [w22 w24] -> w8
      event Panel Close? {
        n121 = event-data() -> ()  [unwired: 1 in, 1 out]
        n122 = event-data("Discard?"=TRUE) -> ()  [unwired: 1 in, 1 out]
        n123 = call <vilib>:"Add State(s) to Queue__JKI_lib_State_Machine.vi"("State(s) in Front (\"\")"="Macro: Exit", "State(s) in (\"\")"=w23) -> ("States Out"=w22:string)  [unwired: 13 in]
      }
      event Timeout {
        n124 = event-data() -> ()  [unwired: 1 in, 1 out]
      }
    }
  }
  n125 = control-ref of="Current VI Reference"() -> (w1:refnum<vi>)
  n126 = call <vilib>:"Clear Errors.vi"("error in (no error)"=w2) -> ("error out"=w5:errorcluster)  [unwired: 5 in, 1 out]
  n127 = call "Close Caller FP if In LabVIEW folder.vi"("reference"=w1, "error in (no error)"=w5) -> ("error out"=w6:errorcluster)  [unwired: 9 in]
  n128 = call <vilib>:"Clear Errors.vi"("error in (no error)"=w6) -> ()  [unwired: 5 in, 2 out]
